vi "Variant to 2D Double Array.vi"(7 "Transpose?":bool, 8 "error in":errorcluster, 11 "Variant":variant) -> (0 "error out":errorcluster, 3 "2D Array":dbl[][](array[numeric]))   [LabVIEW 2018, in "Generic Optimization Actor.lvlib" / "Generic Optimization.lvclass"]
uses:
  Generic Optimization.lvclass
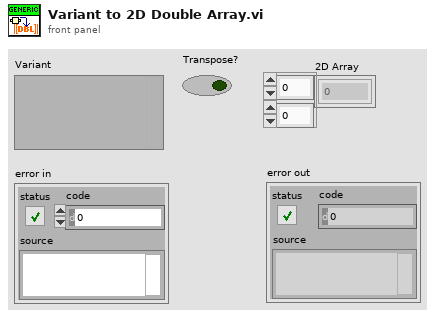
[diagram p1: front panel]
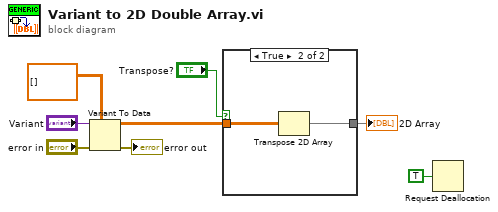
[diagram p0: block diagram]
diagram:
  n1 = Variant To Data(error in="error in", type=dbl[][] [], Variant="Variant") -> (data=w7:dbl[][], error out=→"error out":errorcluster)
  n2 = case shown="True" "Transpose?" {
    tunnel: w7 -> [w9 w11]
    tunnel: [w9 w10] -> w3
    frame False {
    }
    frame True {
      n3 = Transpose 2D Array(2D array=w11) -> (transposed array=w10:dbl[][])
    }
  }
  "2D Array" <- w3
  n4 = Request Deallocation(TRUE ("flag")) -> ()
